vi "Turn Vision - late friday.vi"(0 "Angle from camera":dbl, 1 "AUTO TURN":bool, 5 "From Current Pitch Positon":dbl, 7 "From Joystick V Align":dbl, 9 "Angle Gyro":dbl, 10 "True from shooter":bool, 11 "From joystick Right drive":dbl, 12 "From joystick left drive":dbl) -> (4 "To Left Drive":dbl, 6 "To Corrected Pitch":dbl, 8 "To Joystick V Align":dbl, 14 "True to shooter":bool, 15 "To Right Drive":dbl)   [LabVIEW 2015]
uses:
  <vilib>/Rock Robotics/Network Tables/NT Read Number.vi
  <vilib>/Rock Robotics/Network Tables/NT Read Boolean.vi
  <vilib>/Rock Robotics/Network Tables/NT Write Boolean.vi
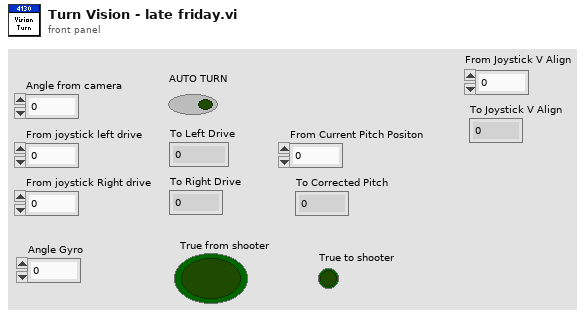
[diagram p1: front panel]
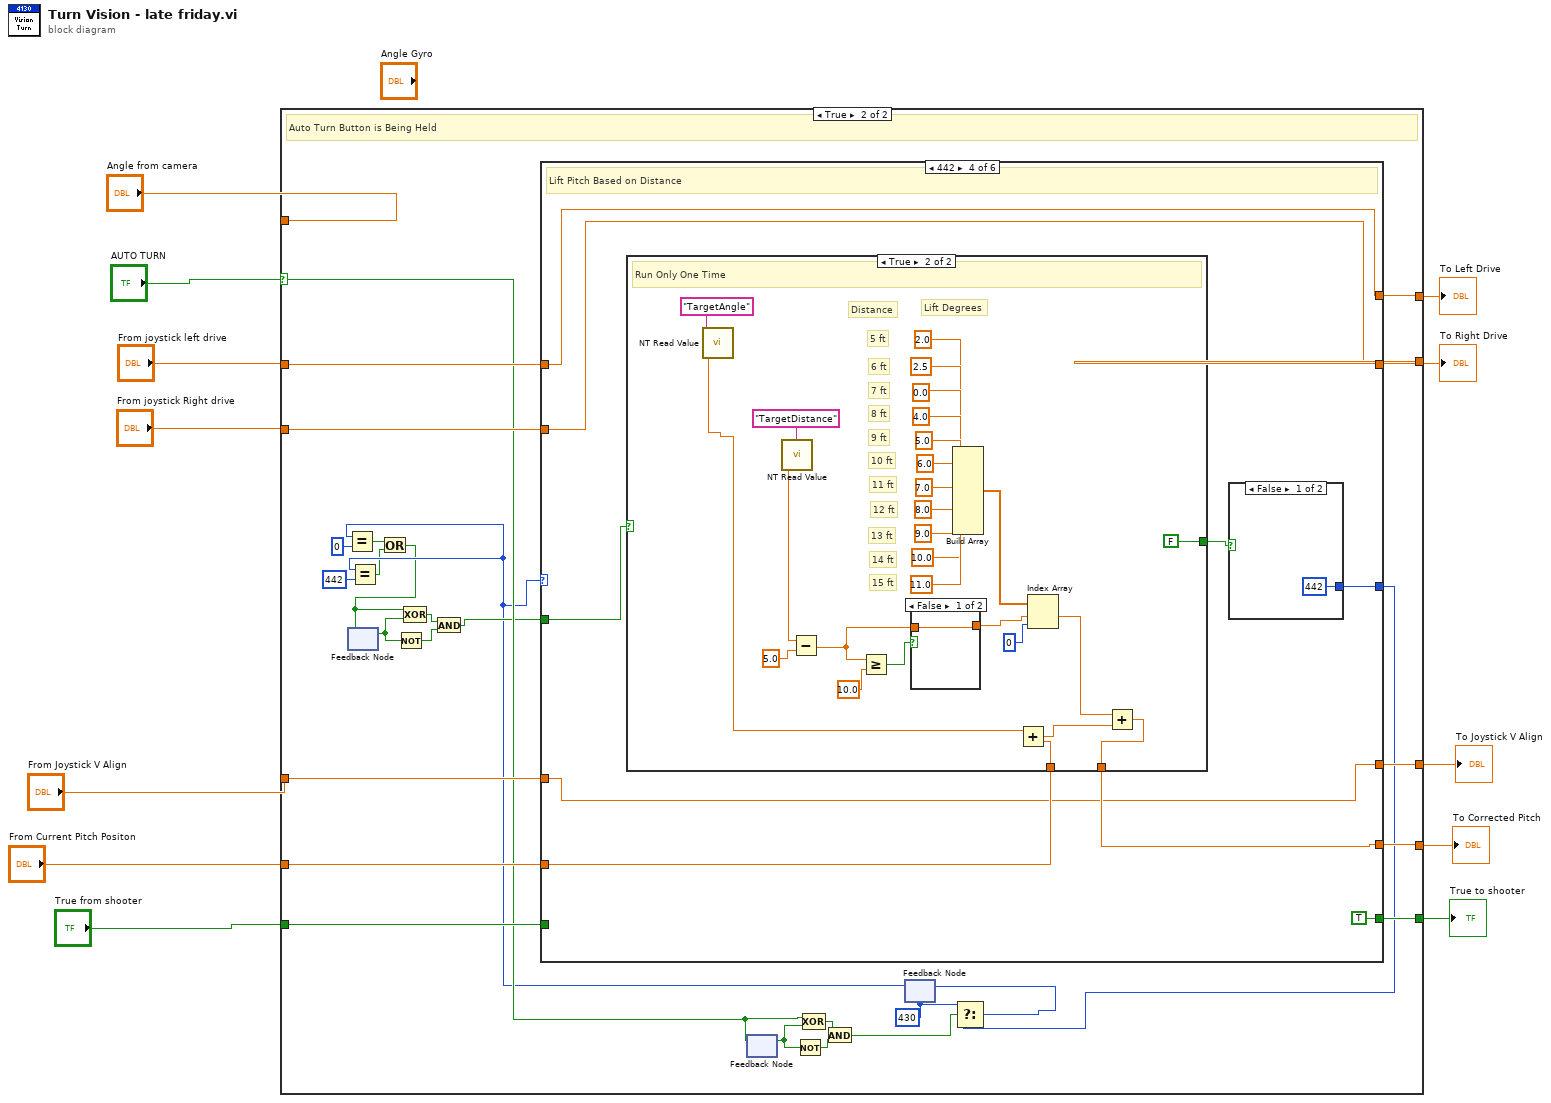
[diagram p0: block diagram]
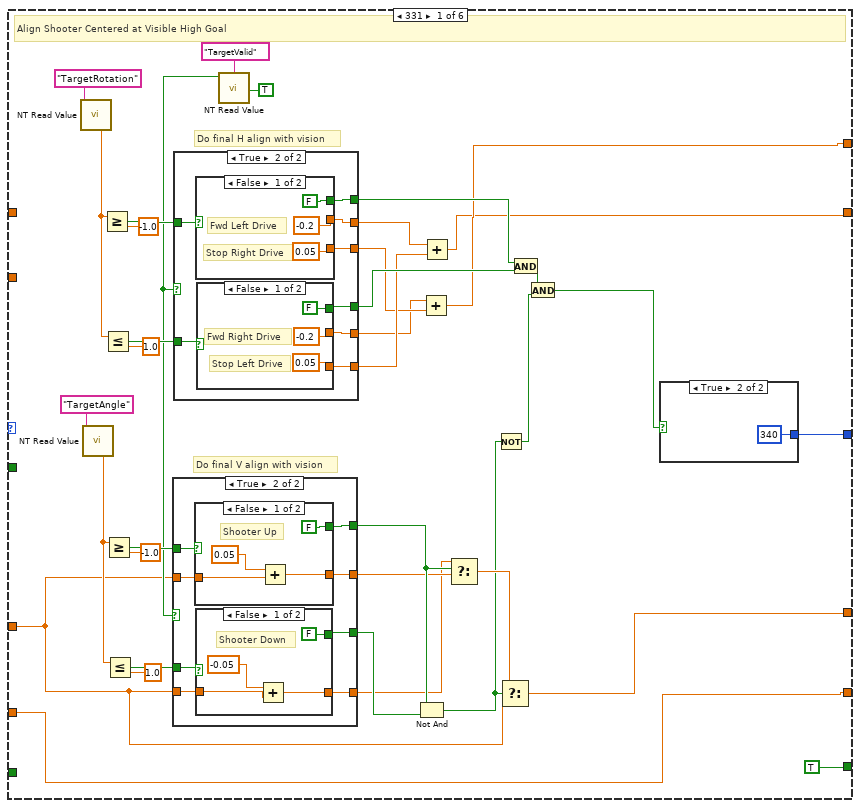
[diagram p3: hidden frame]
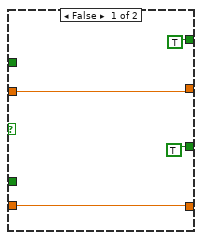
[diagram p4: hidden frame]
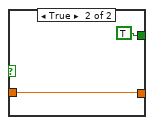
[diagram p5: hidden frame]
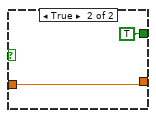
[diagram p6: hidden frame]
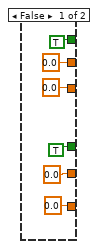
[diagram p7: hidden frame]
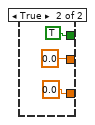
[diagram p8: hidden frame]
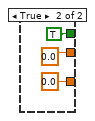
[diagram p9: hidden frame]
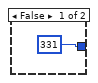
[diagram p10: hidden frame]
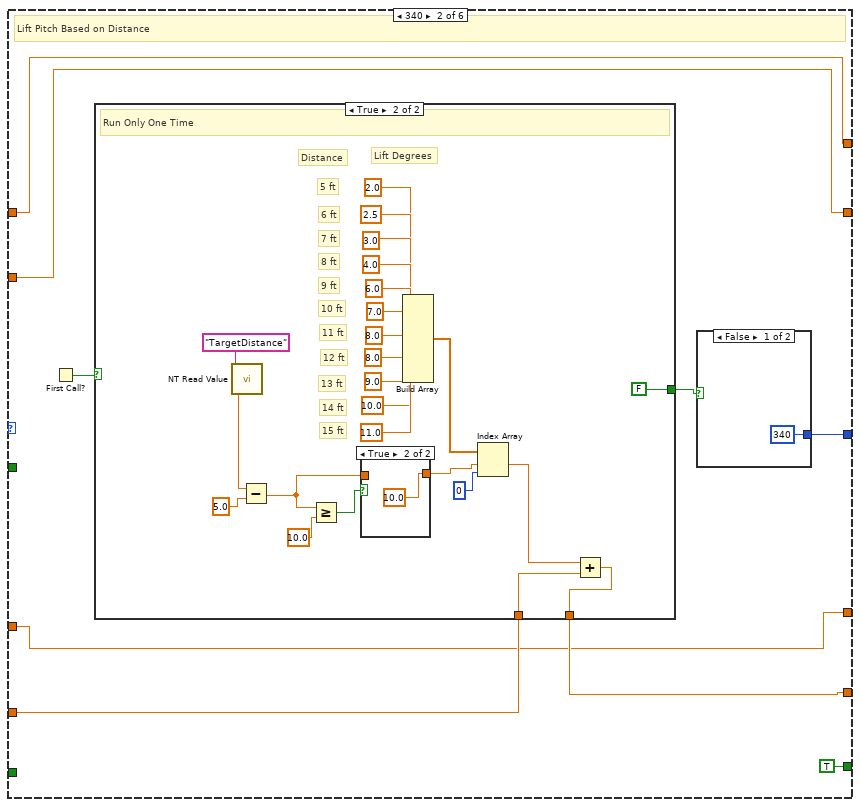
[diagram p11: hidden frame]
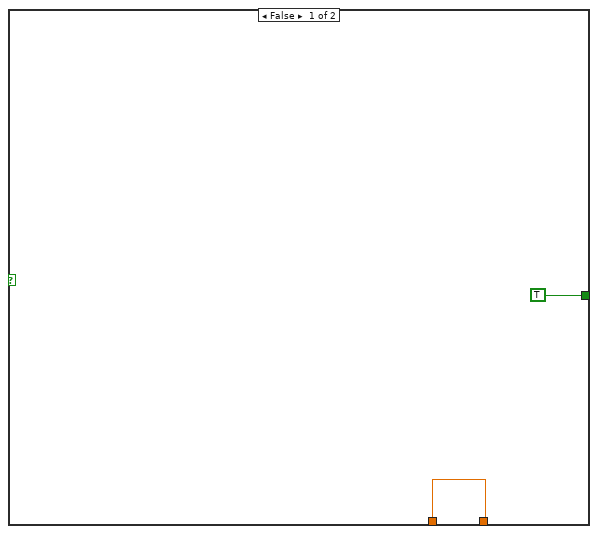
[diagram p12: hidden frame]
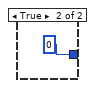
[diagram p14: hidden frame]
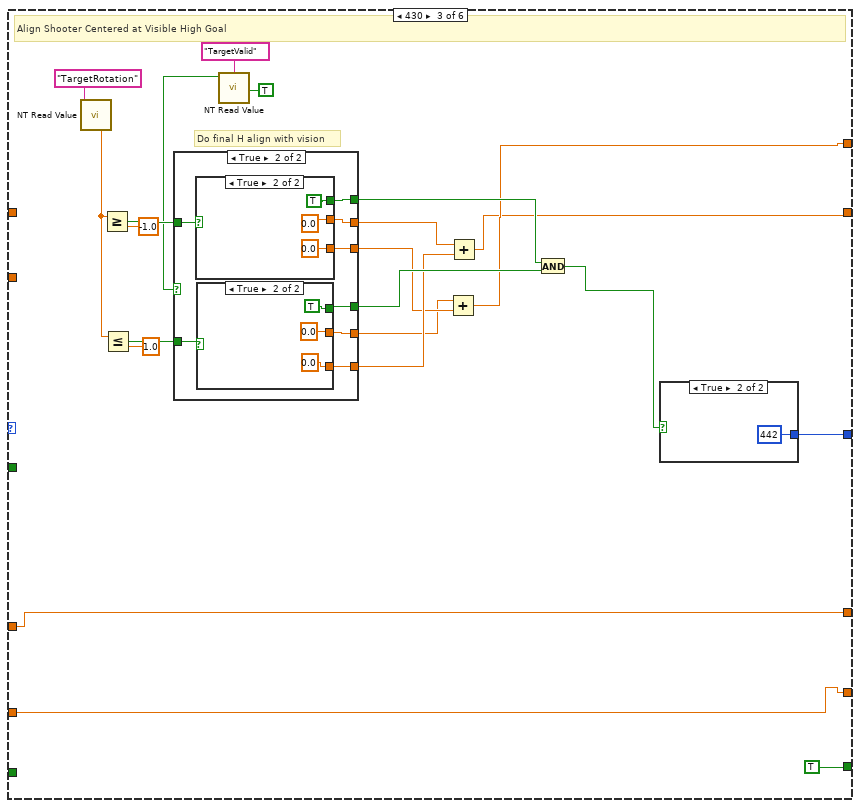
[diagram p15: hidden frame]
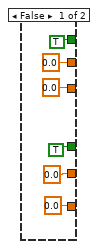
[diagram p16: hidden frame]
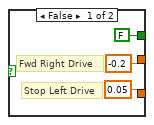
[diagram p17: hidden frame]
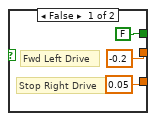
[diagram p18: hidden frame]
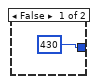
[diagram p19: hidden frame]
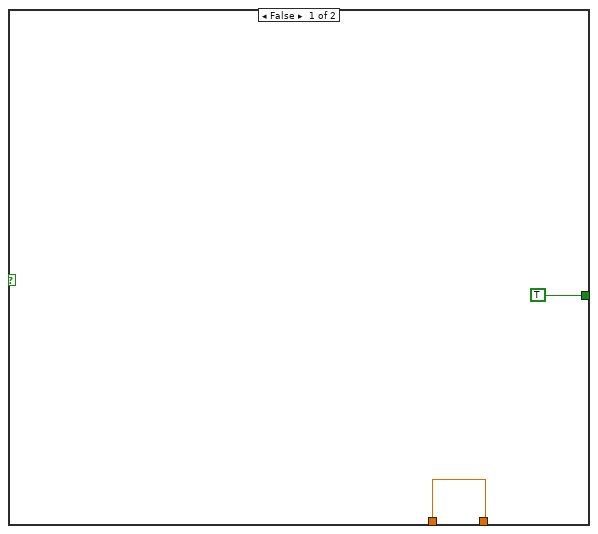
[diagram p20: hidden frame]
diagram:
  n1 = case shown="True" "AUTO TURN" {
    selector: "AUTO TURN" -> [_ w29]
    tunnel: "From joystick Right drive" -> [w17 w40]
    tunnel: "From joystick left drive" -> [w16 w41]
    tunnel: "Angle from camera" -> [_ _]
    tunnel: [w17 w44] -> w11
    tunnel: [w16 w45] -> w12
    tunnel: "From Current Pitch Positon" -> [w15 w43]
    tunnel: [w15 w42] -> w5
    tunnel: "True from shooter" -> [w14 w39]
    tunnel: [w14 w38] -> w3
    tunnel: "From Joystick V Align" -> [w13 w37]
    tunnel: [w13 w36] -> w1
    frame False {
      # "Auto Turn is NOT Pressesd"
    }
    frame True {
      w33 = i64 430 ("milliseconds to wait")
      # "Auto Turn Button is Being Held"
      n2 = feedback #1() -> (w26:bool)  [unwired: 1 in]
      n3 = Not(x=w26) -> (.not. x?=w24:bool)
      n4 = feedback #2() -> (w30:bool)  [unwired: 1 in]
      n5 = feedback-in #2(w29) -> ()
      n6 = Not(x=w30) -> (.not. x?=w32:bool)
      n7 = Compound Arithmetic op=XOR(w29, w30) -> (w31:bool)
      n8 = And(x=w31, y=w32) -> (x .and. y?=w28:bool)
      n9 = feedback #3(w33) -> (w21:i64)
      n10 = Equal?(x=w21, y=i64 0) -> (x = y?=w18:bool)
      n11 = Equal?(x=w21, y=i64 442) -> (x = y?=w19:bool)
      n12 = Or(x=w18, y=w19) -> (x .or. y?=w20:bool)
      n13 = feedback-in #1(w20) -> ()
      n14 = Compound Arithmetic op=XOR(w20, w26) -> (w25:bool)
      n15 = And(x=w25, y=w24) -> (x .and. y?=w23:bool)
      n16 = case shown="442" w21 {
        tunnel: [w82 w141 w195 w230 w268 i64 0 ("milliseconds to wait")] -> w35
        tunnel: [w51 w143 w179 w232 w270 w404] -> w45
        tunnel: [w50 w142 w178 w231 w269 w403] -> w44
        tunnel: w43 -> [w46 w138 w174 w228 w296 w402]
        tunnel: [w46 w139 w174 w229 w272 w402] -> w42
        tunnel: w41 -> [_ w143 _ w232 w270 w404]
        tunnel: w40 -> [_ w142 _ w231 w269 w403]
        tunnel: w39 -> [_ _ _ _ _ w401]
        tunnel: [TRUE TRUE ("True from shooter") TRUE TRUE ("True from shooter") w271 w401] -> w38
        tunnel: w37 -> [w48 w135 w175 w225 w297 w400]
        tunnel: [w47 w135 w175 w225 w297 w400] -> w36
        tunnel: w23 -> [_ _ _ w224 _ w399]
        frame 331 {
          # "Do final V align with vision"
          # "Do final H align with vision"
          # "Align Shooter Centered at Visible High Goal"
          n17 = call-poly <vilib>:"NT Read Value.vi"("Name"="TargetRotation") -> ("Numeric"=w77:dbl)  [unwired: 9 in, 1 out]
          n18 = call-poly <vilib>:"NT Read Value.vi"("Name"="TargetAngle") -> ("Numeric"=w64:dbl)  [unwired: 9 in, 1 out]
          n19 = Greater Or Equal?(x=w77, y=-1.0) -> (x >= y?=w73:bool)
          n20 = Less Or Equal?(x=w77, y=1.0) -> (x <= y?=w72:bool)
          n21 = Greater Or Equal?(x=w64, y=-1.0) -> (x >= y?=w65:bool)
          n22 = Less Or Equal?(x=w64, y=1.0) -> (x <= y?=w66:bool)
          n23 = call-poly <vilib>:"NT Read Value.vi"("Default Value"=TRUE, "Name"="TargetValid") -> ("Boolean"=w60:bool)  [unwired: 8 in, 1 out]
          n24 = case shown="True" w60 {
            tunnel: [TRUE w94] -> w58
            tunnel: w65 -> [_ w93]
            tunnel: w66 -> [_ w92]
            tunnel: [TRUE w91] -> w59
            tunnel: [w84 w90] -> w57
            tunnel: [w83 w89] -> w55
            tunnel: w48 -> [w84 w88]
            tunnel: w48 -> [w83 w87]
            frame False {
            }
            frame True {
              n25 = case shown="False" w93 {
                tunnel: [FALSE TRUE] -> w94
                tunnel: [w103 w105] -> w90
                tunnel: w88 -> [w102 w105]
                frame False {
                  # "Shooter Up"
                  n26 = Add(x=0.05 ("y"), y=w102) -> (x+y=w103:dbl)
                }
                frame True {
                }
              }
              n27 = case shown="False" w92 {
                tunnel: [FALSE TRUE] -> w91
                tunnel: [w96 w99] -> w89
                tunnel: w87 -> [w95 w99]
                frame False {
                  # "Shooter Down"
                  n28 = Add(x=-0.05 ("y"), y=w95) -> (x+y=w96:dbl)
                }
                frame True {
                }
              }
            }
          }
          n29 = case shown="True" w60 {
            tunnel: [TRUE w120] -> w74
            tunnel: w73 -> [_ w119]
            tunnel: w72 -> [_ w118]
            tunnel: [TRUE w117] -> w71
            tunnel: [0.0 ("y") w116] -> w68
            tunnel: [0.0 ("y") w115] -> w67
            tunnel: [0.0 ("y") w114] -> w69
            tunnel: [0.0 ("y") w113] -> w70
            frame False {
            }
            frame True {
              n30 = case shown="False" w119 {
                tunnel: [-0.2 ("y") 0.0 ("y")] -> w115
                tunnel: [FALSE TRUE] -> w120
                tunnel: [0.05 ("y") 0.0 ("y")] -> w114
                frame False {
                  # "Fwd Left Drive"
                  # "Stop Right Drive"
                }
                frame True {
                }
              }
              n31 = case shown="False" w118 {
                tunnel: [-0.2 ("y") 0.0 ("y")] -> w116
                tunnel: [FALSE TRUE] -> w117
                tunnel: [0.05 ("y") 0.0 ("y")] -> w113
                frame False {
                  # "Fwd Right Drive"
                  # "Stop Left Drive"
                }
                frame True {
                }
              }
            }
          }
          n32 = Not And(1:w59, 2:w58) -> (0:w52:bool)
          n33 = Add(x=w68, y=w69) -> (x+y=w51:dbl)
          n34 = Add(x=w67, y=w70) -> (x+y=w50:dbl)
          n35 = Select(t=w55, s=w58, f=w57) -> (s? t:f=w56:dbl)
          n36 = Not(x=w52) -> (.not. x?=w53:bool)
          n37 = Select(t=w56, s=w52, f=w48) -> (s? t:f=w47:dbl)
          n38 = And(x=w74, y=w71) -> (x .and. y?=w81:bool)
          n39 = And(x=w81, y=w53) -> (x .and. y?=w54:bool)
          n40 = case shown="True" w54 {
            tunnel: [i64 331 ("milliseconds to wait") i64 340 ("milliseconds to wait")] -> w82
            frame False {
            }
            frame True {
            }
          }
        }
        frame 340 {
          # "Lift Pitch Based on Distance"
          n41 = First Call?() -> (First Call?: T/F=w140:bool)
          n42 = case shown="True" w140 {
            tunnel: [w144 w152] -> w139
            tunnel: w138 -> [w144 w151]
            tunnel: [TRUE FALSE] -> w137
            frame False {
            }
            frame True {
              # "15 ft"
              # "14 ft"
              # "13 ft"
              # "12 ft"
              # "11 ft"
              # "10 ft"
              # "9 ft"
              # "8 ft"
              # "7 ft"
              # "6 ft"
              # "5 ft"
              # "Lift Degrees"
              # "Distance"
              # "Run Only One Time"
              n43 = call-poly <vilib>:"NT Read Value.vi"("Name"="TargetDistance") -> ("Numeric"=w157:dbl)  [unwired: 9 in, 1 out]
              n44 = Subtract(x=w157, y=5.0) -> (x-y=w147:dbl)
              n45 = Greater Or Equal?(x=w147, y=10.0) -> (x >= y?=w149:bool)
              n46 = case shown="True" w149 {
                tunnel: [w170 10.0 ("y")] -> w148
                tunnel: w147 -> [w170 _]
                frame False {
                }
                frame True {
                }
              }
              n47 = Build Array(2.0 ("element"), 2.5 ("element"), 3.0 ("element"), 4.0 ("element"), 6.0 ("element"), 7.0 ("element"), 8.0 ("element"), 8.0 ("element"), 9.0 ("element"), 10.0 ("element"), 11.0 ("element")) -> (w155:dbl[])
              n48 = Index Array(array=w155, index #1=w148, index #2=0 ("index")) -> (element #1=w153:dbl)  [unwired: 1 out]
              n49 = Add(x=w153, y=w151) -> (x+y=w152:dbl)
            }
          }
          n50 = case shown="False" w137 {
            tunnel: [i64 340 ("milliseconds to wait") i64 0 ("milliseconds to wait")] -> w141
            frame False {
            }
            frame True {
            }
          }
        }
        frame 430 {
          # "Do final H align with vision"
          # "Align Shooter Centered at Visible High Goal"
          n51 = call-poly <vilib>:"NT Read Value.vi"("Name"="TargetRotation") -> ("Numeric"=w191:dbl)  [unwired: 9 in, 1 out]
          n52 = Greater Or Equal?(x=w191, y=-1.0) -> (x >= y?=w187:bool)
          n53 = Less Or Equal?(x=w191, y=1.0) -> (x <= y?=w186:bool)
          n54 = call-poly <vilib>:"NT Read Value.vi"("Default Value"=TRUE, "Name"="TargetValid") -> ("Boolean"=w180:bool)  [unwired: 8 in, 1 out]
          n55 = case shown="True" w180 {
            tunnel: [TRUE w209] -> w188
            tunnel: w187 -> [_ w208]
            tunnel: w186 -> [_ w207]
            tunnel: [TRUE w206] -> w185
            tunnel: [0.0 ("y") w205] -> w182
            tunnel: [0.0 ("y") w204] -> w181
            tunnel: [0.0 ("y") w203] -> w183
            tunnel: [0.0 ("y") w202] -> w184
            frame False {
            }
            frame True {
              n56 = case shown="True" w208 {
                tunnel: [-0.2 ("y") 0.0 ("y")] -> w204
                tunnel: [FALSE TRUE] -> w209
                tunnel: [0.05 ("y") 0.0 ("y")] -> w203
                frame False {
                  # "Fwd Left Drive"
                  # "Stop Right Drive"
                }
                frame True {
                }
              }
              n57 = case shown="True" w207 {
                tunnel: [-0.2 ("y") 0.0 ("y")] -> w205
                tunnel: [FALSE TRUE] -> w206
                tunnel: [0.05 ("y") 0.0 ("y")] -> w202
                frame False {
                  # "Fwd Right Drive"
                  # "Stop Left Drive"
                }
                frame True {
                }
              }
            }
          }
          n58 = Add(x=w182, y=w183) -> (x+y=w179:dbl)
          n59 = Add(x=w181, y=w184) -> (x+y=w178:dbl)
          n60 = And(x=w188, y=w185) -> (x .and. y?=w176:bool)
          n61 = case shown="True" w176 {
            tunnel: [i64 430 ("milliseconds to wait") i64 442 ("milliseconds to wait")] -> w195
            frame False {
            }
            frame True {
            }
          }
        }
        frame 442 {
          # "Lift Pitch Based on Distance"
          n62 = case shown="True" w224 {
            tunnel: [w233 w244] -> w229
            tunnel: w228 -> [w233 w237]
            tunnel: [TRUE FALSE] -> w227
            frame False {
            }
            frame True {
              # "15 ft"
              # "14 ft"
              # "13 ft"
              # "12 ft"
              # "11 ft"
              # "10 ft"
              # "9 ft"
              # "8 ft"
              # "7 ft"
              # "6 ft"
              # "5 ft"
              # "Lift Degrees"
              # "Distance"
              # "Run Only One Time"
              n63 = call-poly <vilib>:"NT Read Value.vi"("Name"="TargetAngle") -> ("Numeric"=w235:dbl)  [unwired: 9 in, 1 out]
              n64 = call-poly <vilib>:"NT Read Value.vi"("Name"="TargetDistance") -> ("Numeric"=w249:dbl)  [unwired: 9 in, 1 out]
              n65 = Subtract(x=w249, y=5.0) -> (x-y=w240:dbl)
              n66 = Greater Or Equal?(x=w240, y=10.0) -> (x >= y?=w242:bool)
              n67 = case shown="False" w242 {
                tunnel: [w262 10.0 ("y")] -> w241
                tunnel: w240 -> [w262 _]
                frame False {
                }
                frame True {
                }
              }
              n68 = Build Array(2.0 ("element"), 2.5 ("element"), 0.0 ("element"), 4.0 ("element"), 5.0 ("element"), 6.0 ("element"), 7.0 ("element"), 8.0 ("element"), 9.0 ("element"), 10.0 ("element"), 11.0 ("element")) -> (w247:dbl[])
              n69 = Add(x=w235, y=w237) -> (x+y=w236:dbl)
              n70 = Index Array(array=w247, index #1=w241, index #2=0 ("index")) -> (element #1=w245:dbl)  [unwired: 1 out]
              n71 = Add(x=w245, y=w236) -> (x+y=w244:dbl)
            }
          }
          n72 = case shown="False" w227 {
            tunnel: [i64 442 ("milliseconds to wait") i64 0 ("milliseconds to wait")] -> w230
            frame False {
            }
            frame True {
            }
          }
        }
        frame 500 {
          n73 = call-poly <vilib>:"NT Read Value.vi"("Name"="TargetDistance") -> ("Numeric"=w286:dbl)  [unwired: 9 in, 1 out]
          n74 = Equal?(x=w286, y=5.0) -> (x = y?=w283:bool)
          n75 = Equal?(x=w286, y=6.0) -> (x = y?=w282:bool)
          n76 = Equal?(x=w286, y=7.0) -> (x = y?=w281:bool)
          n77 = Equal?(x=w286, y=8.0) -> (x = y?=w280:bool)
          n78 = Equal?(x=w286, y=9.0) -> (x = y?=w279:bool)
          n79 = Equal?(x=w286, y=10.0) -> (x = y?=w278:bool)
          n80 = Equal?(x=w286, y=11.0) -> (x = y?=w277:bool)
          n81 = Equal?(x=w286, y=12.0) -> (x = y?=w276:bool)
          n82 = Equal?(x=w286, y=13.0) -> (x = y?=w275:bool)
          n83 = Equal?(x=w286, y=14.0) -> (x = y?=w274:bool)
          n84 = Equal?(x=w286, y=15.0) -> (x = y?=w273:bool)
          n85 = case shown="False" w283 {
            tunnel: w296 -> [_ _]
            tunnel: w282 -> [w311 _]
            tunnel: w281 -> [w310 _]
            tunnel: w280 -> [w309 _]
            tunnel: w279 -> [w308 _]
            tunnel: w278 -> [w307 _]
            tunnel: w277 -> [w306 _]
            tunnel: w276 -> [w305 _]
            tunnel: w275 -> [w304 _]
            tunnel: w274 -> [w303 _]
            tunnel: w273 -> [w302 _]
            tunnel: [w301 52.0 ("y")] -> w272
            tunnel: [w300 TRUE] -> w271
            frame False {
              n86 = case shown="False" w311 {
                tunnel: w310 -> [w322 _]
                tunnel: w309 -> [w321 _]
                tunnel: w308 -> [w320 _]
                tunnel: w307 -> [w319 _]
                tunnel: w306 -> [w318 _]
                tunnel: w305 -> [w317 _]
                tunnel: w304 -> [w316 _]
                tunnel: w303 -> [w315 _]
                tunnel: w302 -> [w314 _]
                tunnel: [w313 50.0 ("y")] -> w301
                tunnel: [w312 TRUE] -> w300
                frame False {
                  n87 = case shown="False" w322 {
                    tunnel: w321 -> [w332 _]
                    tunnel: w320 -> [w331 _]
                    tunnel: w319 -> [w330 _]
                    tunnel: w318 -> [w329 _]
                    tunnel: w317 -> [w328 _]
                    tunnel: w316 -> [w327 _]
                    tunnel: w315 -> [w326 _]
                    tunnel: w314 -> [w325 _]
                    tunnel: [w324 48.0 ("y")] -> w313
                    tunnel: [w323 TRUE] -> w312
                    frame False {
                      n88 = case shown="False" w332 {
                        tunnel: w331 -> [w341 _]
                        tunnel: w330 -> [w340 _]
                        tunnel: w329 -> [w339 _]
                        tunnel: w328 -> [w338 _]
                        tunnel: w327 -> [w337 _]
                        tunnel: w326 -> [w336 _]
                        tunnel: w325 -> [w335 _]
                        tunnel: [w334 46.0 ("y")] -> w324
                        tunnel: [w333 TRUE] -> w323
                        frame False {
                          n89 = case shown="False" w341 {
                            tunnel: w340 -> [w349 _]
                            tunnel: w339 -> [w348 _]
                            tunnel: w338 -> [w347 _]
                            tunnel: w337 -> [w346 _]
                            tunnel: w336 -> [w345 _]
                            tunnel: w335 -> [w344 _]
                            tunnel: [w343 44.0 ("y")] -> w334
                            tunnel: [w342 TRUE] -> w333
                            frame False {
                              n90 = case shown="False" w349 {
                                tunnel: w348 -> [w356 _]
                                tunnel: w347 -> [w355 _]
                                tunnel: w346 -> [w354 _]
                                tunnel: w345 -> [w353 _]
                                tunnel: w344 -> [w352 _]
                                tunnel: [w351 42.0 ("y")] -> w343
                                tunnel: [w350 TRUE] -> w342
                                frame False {
                                n91 = case shown="False" w356 {
                                tunnel: w355 -> [w362 _]
                                tunnel: w354 -> [w361 _]
                                tunnel: w353 -> [w360 _]
                                tunnel: w352 -> [w359 _]
                                tunnel: [w358 40.0 ("y")] -> w351
                                tunnel: [w357 TRUE] -> w350
                                frame False {
                                n92 = case shown="False" w362 {
                                tunnel: w361 -> [w367 _]
                                tunnel: w360 -> [w366 _]
                                tunnel: w359 -> [w365 _]
                                tunnel: [w364 38.0 ("y")] -> w358
                                tunnel: [w363 TRUE] -> w357
                                frame False {
                                n93 = case shown="False" w367 {
                                tunnel: w366 -> [w371 _]
                                tunnel: w365 -> [w370 _]
                                tunnel: [w369 36.0 ("y")] -> w364
                                tunnel: [w368 TRUE] -> w363
                                frame False {
                                n94 = case shown="False" w371 {
                                tunnel: w370 -> [w374 _]
                                tunnel: [w373 34.0 ("y")] -> w369
                                tunnel: [w372 TRUE] -> w368
                                frame False {
                                n95 = case shown="True" w374 {
                                tunnel: [0.0 ("y") 32.0 ("y")] -> w373
                                tunnel: [FALSE TRUE] -> w372
                                frame False {
                                }
                                frame True {
                                }
                                }
                                }
                                frame True {
                                }
                                }
                                }
                                frame True {
                                }
                                }
                                }
                                frame True {
                                }
                                }
                                }
                                frame True {
                                }
                                }
                                }
                                frame True {
                                }
                              }
                            }
                            frame True {
                            }
                          }
                        }
                        frame True {
                        }
                      }
                    }
                    frame True {
                    }
                  }
                }
                frame True {
                }
              }
            }
            frame True {
            }
          }
          n96 = case shown="False" TRUE {
            tunnel: [i64 500 ("milliseconds to wait") i64 0 ("milliseconds to wait")] -> w268
            frame False {
            }
            frame True {
            }
          }
        }
        frame 0, Default {
          n97 = case shown="True" w399 {
            frame False {
              n98 = call-poly <vilib>:"NT Write Value.vi"("Boolean"=FALSE, "Name"="TargetShootNow") -> ()  [unwired: 9 in, 1 out]
            }
            frame True {
              n99 = call "Elapsed Time2"("Time Target (s)"=2.5) -> ("Time has Elapsed"=w409:bool)  [unwired: 11 in, 7 out]
              n100 = Not(x=w409) -> (.not. x?=w408:bool)
              n101 = call-poly <vilib>:"NT Write Value.vi"("Boolean"=w408, "Name"="TargetShootNow") -> ()  [unwired: 9 in, 1 out]
            }
          }
        }
      }
      n102 = Select(t=w33, s=w28, f=w35) -> (s? t:f=w34:i64)
      n103 = feedback-in #3(w34) -> ()
    }
  }
  "To Left Drive" <- w12
  "To Right Drive" <- w11
  "To Corrected Pitch" <- w5
  "True to shooter" <- w3
  "To Joystick V Align" <- w1
